vi "StartScan.vi"(8 "error in":T1, 11 "State":i32=1) -> (0 "error out":T1)   [LabVIEW 2016]
doc: "Starts ('State' = 1) or stops ('State' = 0) the scanner."
uses:
  Controls/Error_Out.ctl
  Files_ASC500/DLL/ASC500_RemoteControlV27.dll
panel:
  out "mar":i32[](array[numeric])
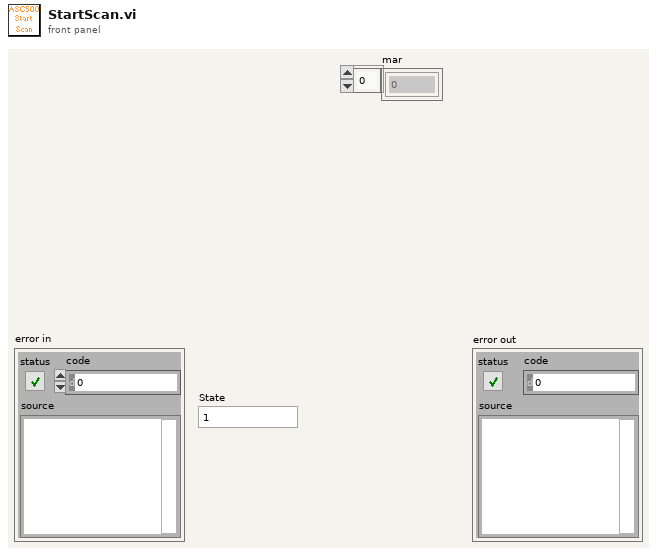
[diagram p1: front panel]
types:
  T1 = typedef "Error_Out.ctl" = errorcluster
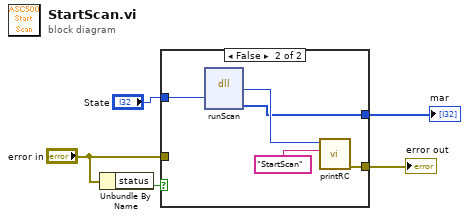
[diagram p0: block diagram]
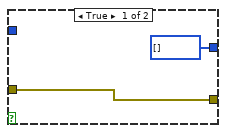
[diagram p2: hidden frame]
diagram:
  n1 = Unbundle By Name("error in") -> ("status"=w5:bool)
  n2 = case shown="False" w5 {
    tunnel: [w7 w11] -> w4
    tunnel: "State" -> [_ w12]
    tunnel: "error in" -> [w7 _]
    tunnel: [i32[] [] ("mar") w8] -> w1
    frame True {
    }
    frame False {
      n3 = dll-call lib="G:/SCMOperations/Share/ELE/Produkt Information/ASC500/04 Remote Control/02 development versions/2018Nov06/Files_ASC500/DLL/ASC500_RemoteControlV27.dll" fn="runScan"("State"=w12) -> ("return type"=w10:i32, "mar"=w8:i32[])  [unwired: 5 in, 2 out]
      n4 = call "printRC.vi"("additional information"="StartScan", "RC"=w10) -> ("error out"=w11:T1)  [unwired: 9 in]
    }
  }
  "error out" <- w4
  "mar" <- w1
